vi "innovation covariance.vi"(7 "R":T1=[[0.1]], 11 "Pk|k-1":T1) -> (2 "S_k array":dbl[][](array[numeric]), 3 "S_k":T1)   [LabVIEW 2016]
uses:
  <vilib>/Analysis/Matrix/Datatypes/RealMatrix.ctl
  <vilib>/Analysis/Matrix/Numeric/Multiply/Multiply - RM,RM.vi
  <vilib>/Analysis/Matrix/Numeric/Add/Add - RM,RM.vi
  <vilib>/Analysis/Matrix/Numeric/Conversions/Matrix To Array - RM.vi
  <vilib>/Analysis/Matrix/NI_Matrix.lvlib
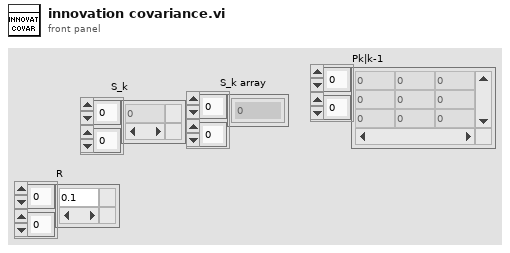
[diagram p1: front panel]
types:
  T1 = typedef "NI_Matrix.lvlib/RealMatrix.ctl" = dbl[][]
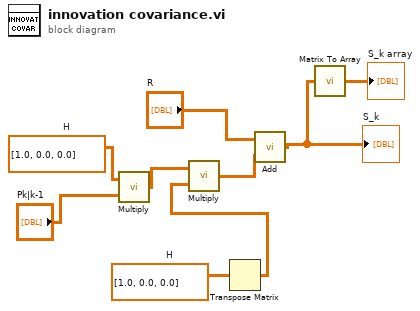
[diagram p0: block diagram]
diagram:
  w2 = T1 [[1.0, 0.0, 0.0]]  # H
  w3 = T1 [[1.0, 0.0, 0.0]]  # H
  n1 = call-poly <vilib>:"Multiply.vi"("Real Matrix B"="Pk|k-1", "Real Matrix A"=w2) -> ("A * B"=w9:T1)
  n2 = Transpose Matrix(1:w3) -> (0:w6:T1)
  n3 = call-poly <vilib>:"Multiply.vi"("Real Matrix B"=w6, "Real Matrix A"=w9) -> ("A * B"=w8:T1)
  n4 = call-poly <vilib>:"Add.vi"("Real Matrix B"=w8, "Real Matrix A"="R") -> ("A + B"=w5:T1)
  "S_k" <- w5
  n5 = call-poly <vilib>:"Matrix To Array.vi"("Real Matrix"=w5) -> ("Real 2D Array"=→"S_k array":dbl[][])
